vi "Untitled 2 (SubVI).vi"(11 "farenheit":dbl) -> (3 "celsius":dbl)   [LabVIEW 2017]
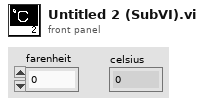
[diagram p1: front panel]
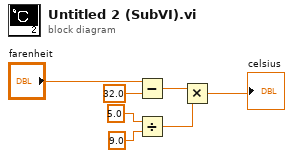
[diagram p0: block diagram]
diagram:
  n1 = Subtract(x="farenheit", y=32.0) -> (x-y=w3:dbl)
  n2 = Divide(x=5.0, y=9.0) -> (x/y=w6:dbl)
  n3 = Multiply(x=w3, y=w6) -> (x*y=→"celsius":dbl)
